vi "GetCompatibleCommands.vi"(0 "Universal Robot in":refnum<class "Universal Robot.lvclass">) -> (14 "Universal Robot Out":refnum<class "Universal Robot.lvclass">, 16 "compatibleCommandList":string[](array[string]), 19 "compatibleCommands":T1[](array[typedef]))   [LabVIEW 2016, in "Universal Robot.lvclass"]
uses:
  Universal Robot.lvclass
  PolyScopeCommand.ctl
  PolyScopeVersion.ctl
  Universal Robot.lvclass/Universal Robot.ctl
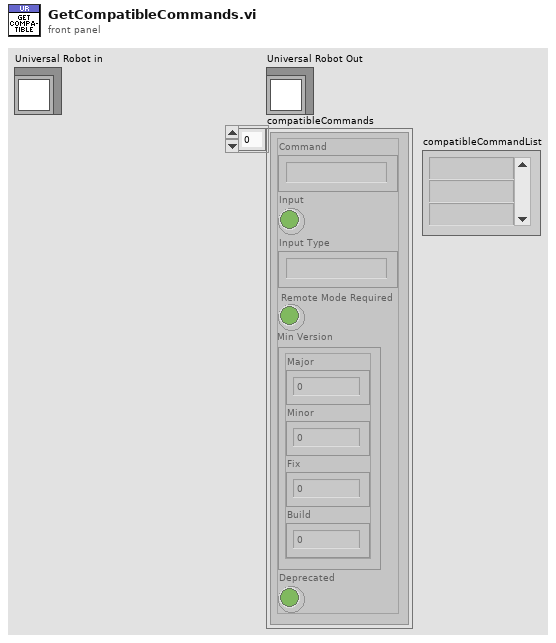
[diagram p1: front panel]
types:
  T1 = typedef "Universal Robot.lvclass/PolyScopeCommand.ctl" = cluster{"Command":string, "Input":bool, "Input Type":string, "Remote Mode Required":bool, "Min Version":T2, "Deprecated":bool}
  T2 = typedef "Universal Robot.lvclass/PolyScopeVersion.ctl" = cluster{"Major":i32, "Minor":i32, "Fix":i32, "Build":i32}
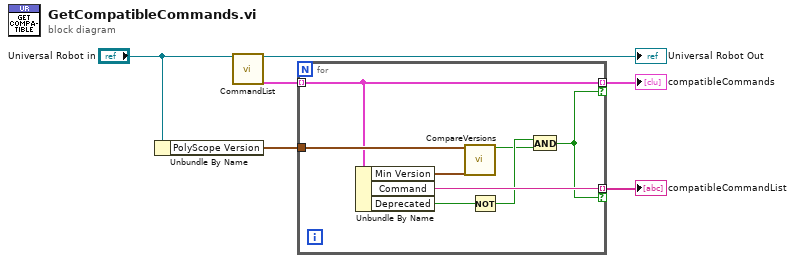
[diagram p0: block diagram]
diagram:
  n1 = Unbundle By Name("Universal Robot in") -> ("PolyScope Version"=w6:T2)
  n2 = call-dynamic "CommandList.vi"("DashboardServer.lvclass"="Universal Robot in") -> ("DashboardServer.lvclass out"=→"Universal Robot Out":refnum<class "Universal Robot.lvclass">, "Compatible Commands"=w1:T1[])  [unwired: 17 in]
  n3 = for {
    tunnel: w1 -> [w12] mode=indexing
    tunnel: w6 -> [w14]
    tunnel: [w12] -> w5 mode=indexing if=w7
    tunnel: [w11] -> w4 mode=indexing if=w7
    n4 = Unbundle By Name(w12) -> ("Min Version"=w13:T2, "Command"=w11:string, "Deprecated"=w10:bool)
    n5 = call "CompareVersions.vi"("robotPolyScopeVersion"=w14, "commandMinVersion"=w13) -> ("compatible"=w8:bool)  [unwired: 17 in]
    n6 = Not(x=w10) -> (.not. x?=w9:bool)
    n7 = And(x=w9, y=w8) -> (x .and. y?=w7:bool)
  }
  "compatibleCommands" <- w5
  "compatibleCommandList" <- w4
